vi "fail display.vi"(1 "P/F":bool[](array[boolean]), 2 "yellow":bool[](array[boolean]), 3 "Multipart board":cluster{"Row":i32, "Colum":i32}={"Row"=8, "Colum"=4}, 4 "colse":refnum<vi>) -> (0 "exit":bool=TRUE)   [LabVIEW 2018]
uses:
  <vilib>/Utility/miscctls.llb/LVBoundsTypeDef.ctl
  <vilib>/Utility/miscctls.llb/LVRowAndColumnTypeDef.ctl
panel:
  out "添加的数组":bool[][](array[boolean])
  out "数组 3":cluster{"Row":i32, "列":i32}[][](array[cluster])
  out "数组 2":cluster{"Row":i32, "列":i32}[](array[cluster])
  in  "F5":bool
  out "显示良品":u32(colorbox)=6618880
  out "显示不良品":u32(colorbox)=16711680
  out "数组":i32[][](array[numeric])
  out "输出簇 2":T1 caption="输出簇"
  out "输出簇":T1
  in  "表格控件":string[][](table)
  # "不良位置显示"
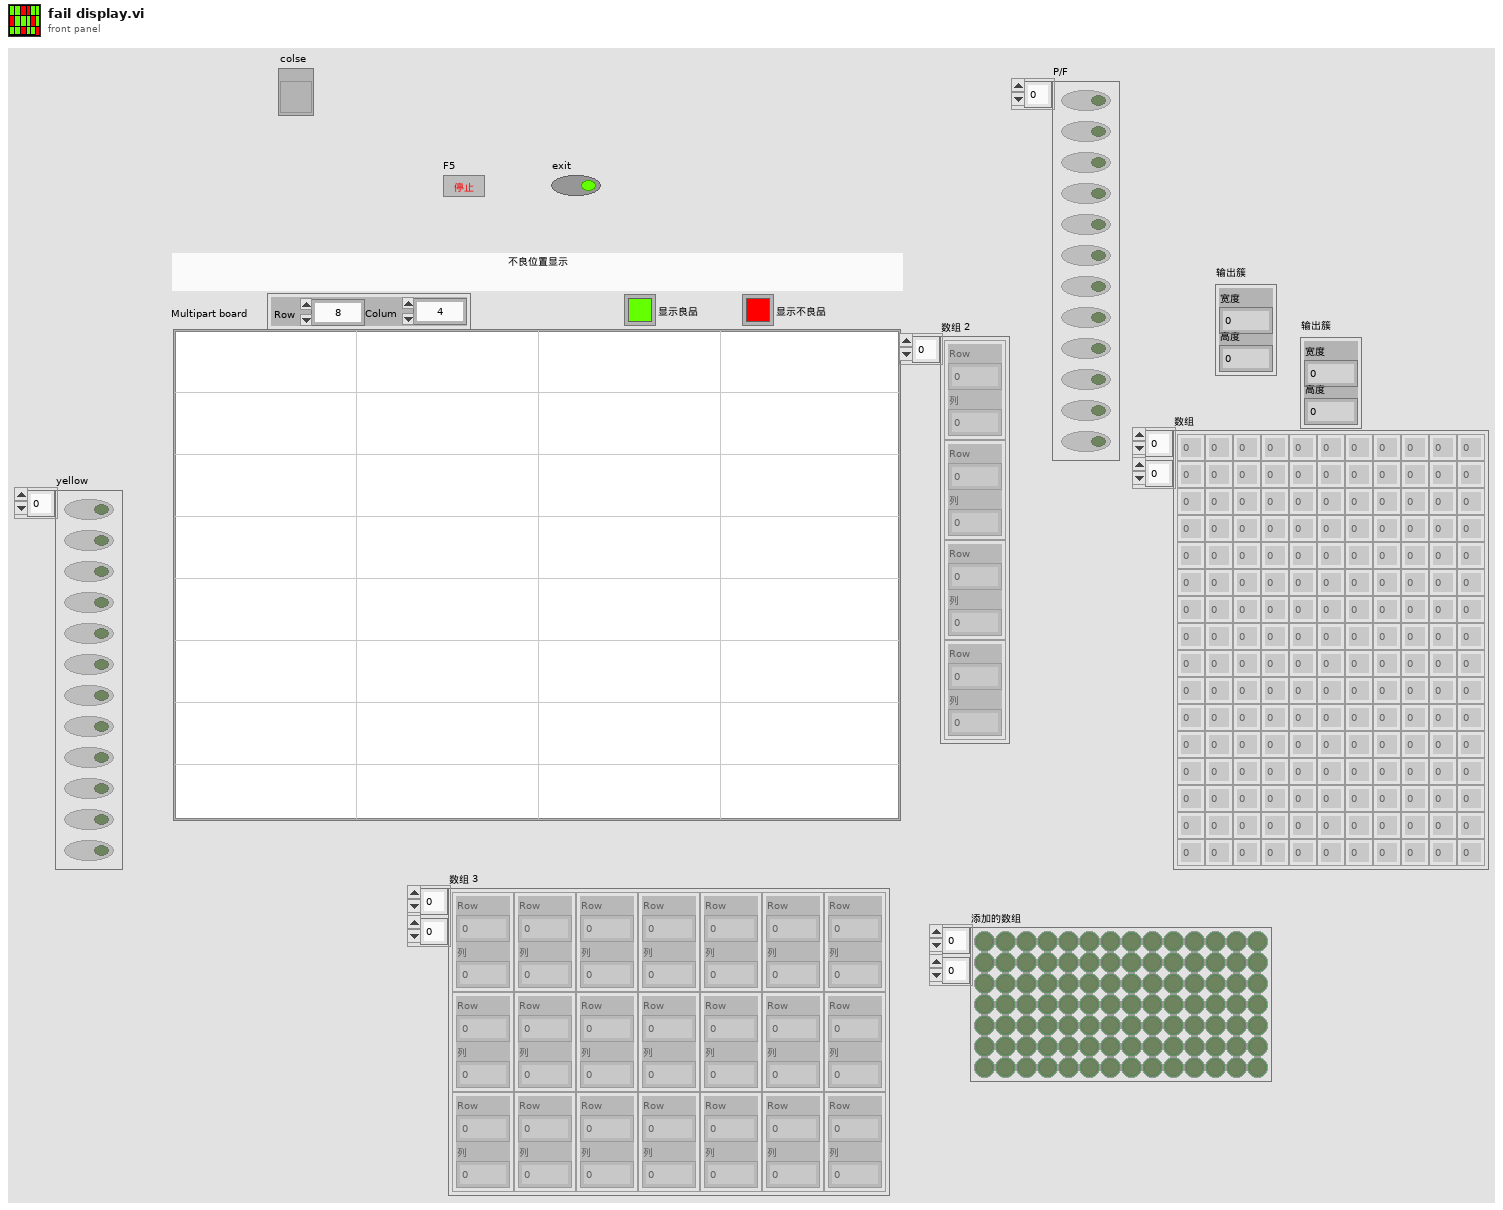
[diagram p1: front panel]
types:
  T1 = typedef "LVBoundsTypeDef.ctl" = cluster{"Width":u32, "Height":u32}
  T2 = typedef "LVRowAndColumnTypeDef.ctl" = cluster{"Row":i32, "Column":i32}
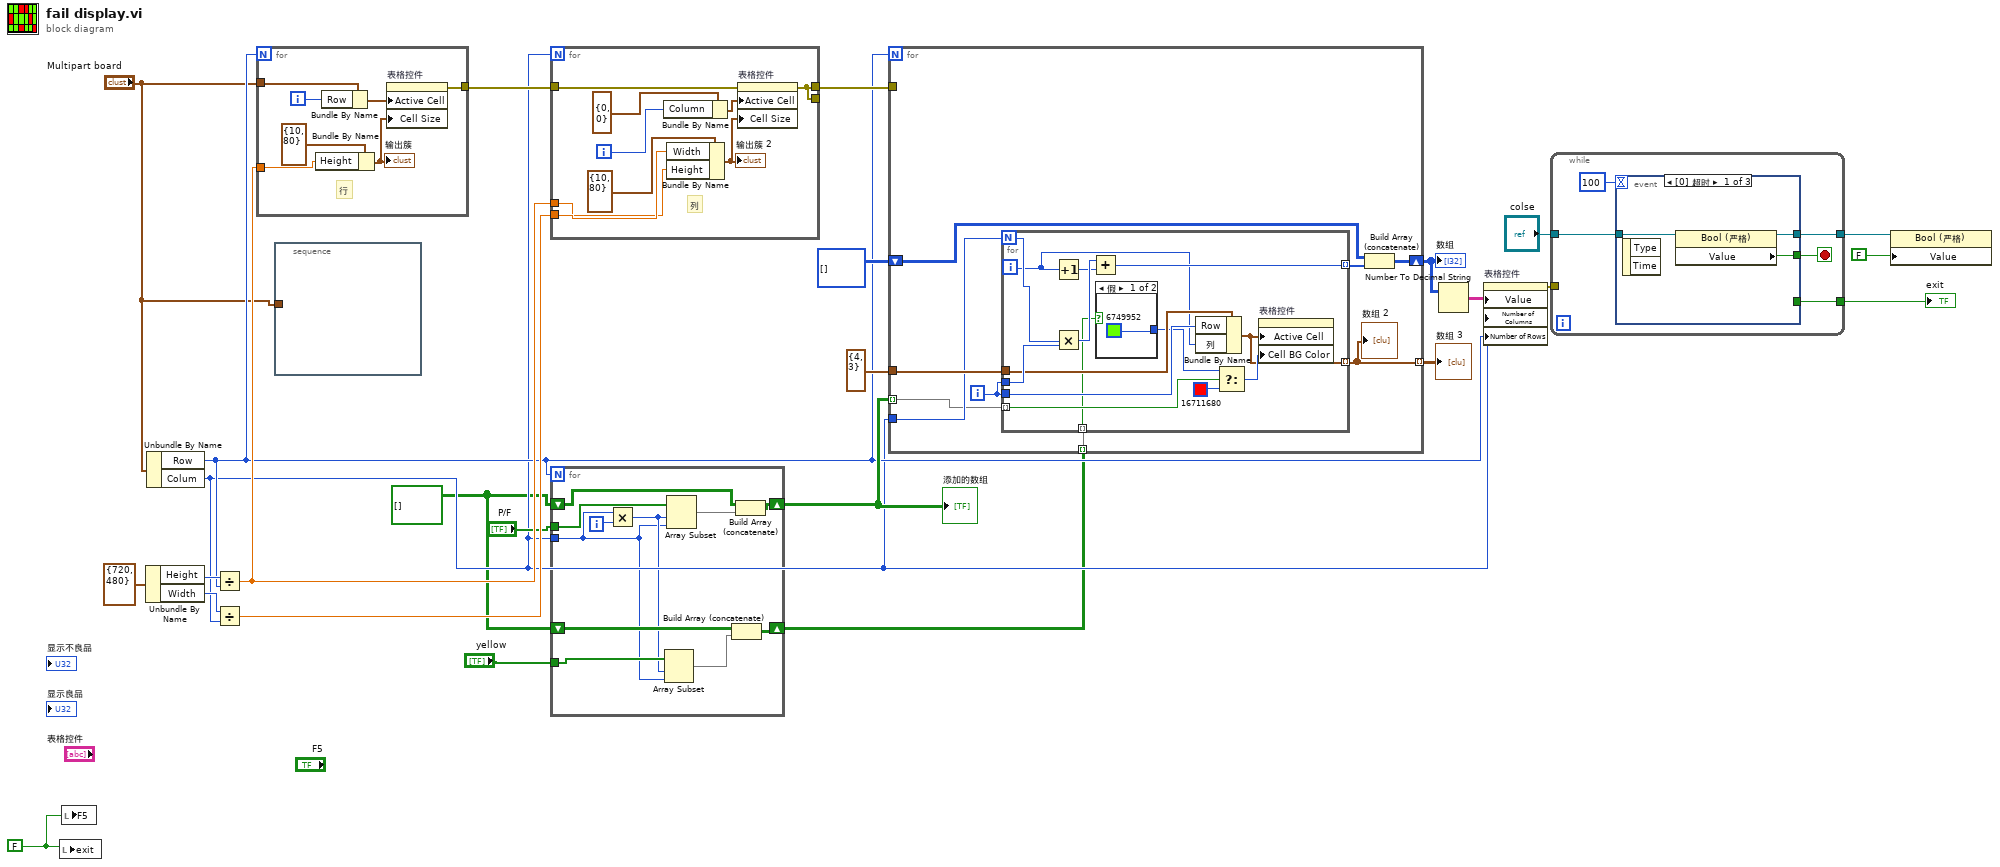
[diagram p0: block diagram]
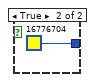
[diagram p2: hidden frame]
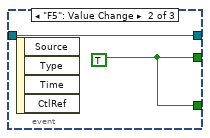
[diagram p3: hidden frame]
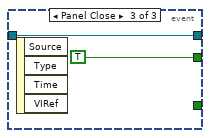
[diagram p4: hidden frame]
diagram:
  w1 = FALSE
  w6 = bool[][] [] ("添加的数组 2")
  n1 = local write "exit"(w1) -> ()
  n2 = local write "F5"(w1) -> ()
  n3 = Unbundle By Name(T1 {"Width"=720, "Height"=480} ("大小")) -> ("Height"=w18:u32, "Width"=w19:u32)
  n4 = Unbundle By Name("Multipart board") -> ("Row"=w9:i32, "Colum"=w8:i32)
  n5 = Divide(x=w18, y=w9) -> (x/y=w21:dbl)
  n6 = Divide(x=w19, y=w8) -> (x/y=w20:dbl)
  n7 = for {
    N: w9 -> [_]
    tunnel: w21 -> [w31]
    tunnel: [w29] -> w22
    tunnel: "Multipart board" -> [w27]
    i -> [w28]
    # "行"
    n8 = Bundle By Name(cluster=T1 {"Width"=10, "Height"=80} ("活动单元格:单元格大小"), "Height"=w31) -> (w30:T1)
    "输出簇" <- w30
    n9 = Bundle By Name(cluster=w27, "Row"=w28) -> (w33:cluster{"Row":i32, "Colum":i32})
    n10 = property on="表格控件" class="Tbl (严格)"("Active Cell"=w33, "Cell Size"=w30) -> (error out=w29:errorcluster)  [unwired: 2 in, 1 out]
  }
  n11 = stacked-sequence {
    tunnel: "Multipart board" -> [_]
    frame #0 {
    }
  }
  n12 = for {
    N: w8 -> [_]
    tunnel: w20 -> [w38]
    tunnel: w21 -> [w36]
    tunnel: w22 -> [w35]
    tunnel: [w34] -> _
    tunnel: [w34] -> w12
    i -> [w41]
    # "列"
    n13 = Bundle By Name(cluster=T2 {"Row"=0, "Column"=0} ("活动单元格:活动单元格"), "Column"=w41) -> (w42:T2)
    n14 = Bundle By Name(cluster=T1 {"Width"=10, "Height"=80} ("活动单元格:单元格大小"), "Width"=w38, "Height"=w36) -> (w37:T1)
    "输出簇 2" <- w37
    n15 = property on="表格控件" class="Tbl (严格)"(error in=w35, "Active Cell"=w42, "Cell Size"=w37) -> (error out=w34:errorcluster)  [unwired: 1 in, 1 out]
  }
  n16 = for {
    N: w9 -> [_]
    shift-right: [w51] -> w10
    shift-left: w6 -> [w52]
    tunnel: "P/F" -> [w53]
    tunnel: w8 -> [w43]
    tunnel: "yellow" -> [w46]
    shift-right: [w47] -> w4
    shift-left: w6 -> [w48]
    i -> [w49]
    n17 = Multiply(x=w43, y=w49) -> (x*y=w44:i32)
    n18 = Array Subset(array=w46, index=w44, length=w43) -> (w45:bool[])
    n19 = Array Subset(array=w53, index=w44, length=w43) -> (w50:bool[])
    n20 = Build Array (concatenate)(w48, w45) -> (w47:bool[][])
    n21 = Build Array (concatenate)(w52, w50) -> (w51:bool[][])
  }
  "添加的数组" <- w10
  n22 = for {
    N: w9 -> [_]
    shift-right: [w61] -> w24
    shift-left: i32[][] [] -> [w62]
    tunnel: w8 -> [w58]
    tunnel: cluster{"Row":i32, "列":i32} {"Row"=4, "列"=3} ("多联板 2") -> [w59]
    tunnel: w10 -> [w56] mode=indexing
    tunnel: [w55] -> w13 mode=indexing
    tunnel: w12 -> [_]
    tunnel: w4 -> [w54] mode=indexing
    i -> [w57]
    n23 = for {
      N: w58 -> [w75]
      tunnel: [w76] -> w60 mode=indexing
      tunnel: w57 -> [w74]
      tunnel: w59 -> [w71]
      tunnel: w57 -> [w69]
      tunnel: w56 -> [w68] mode=indexing
      tunnel: [w67] -> w55 mode=indexing
      tunnel: w54 -> [w63] mode=indexing
      i -> [w65]
      n24 = Increment(x=w65) -> (x+1=w72:i32)
      n25 = Multiply(x=w75, y=w74) -> (x*y=w73:i32)
      n26 = Add(x=w73, y=w72) -> (x+y=w76:i32)
      n27 = case shown="假" w63 {
        tunnel: [u32 6749952 u32 16776704] -> w64
        frame False {
        }
        frame True {
        }
      }
      n28 = Bundle By Name(cluster=w71, "Row"=w69, "列"=w65) -> (w67:cluster{"Row":i32, "列":i32})
      n29 = Select(t=w64, s=w68, f=u32 16711680) -> (s? t:f=w70:u32)
      n30 = property on="表格控件" class="Tbl (严格)"("Active Cell"=w67, "Cell BG Color"=w70) -> ()  [unwired: 2 in, 2 out]
    }
    "数组 2" <- w55
    n31 = Build Array (concatenate)(w62, w60) -> (w61:i32[][])
  }
  "数组" <- w24
  "数组 3" <- w13
  n32 = Number To Decimal String(number=w24) -> (decimal integer string=w25:string[][])  [unwired: 1 out]
  n33 = property on="表格控件" class="Tbl (严格)"("Value"=w25, "Number of Columns"=w8, "Number of Rows"=w9) -> (error out=w16:errorcluster)  [unwired: 2 in, 1 out]
  n34 = while {
    tunnel: "colse" -> [w83]
    tunnel: [w80] -> w14
    tunnel: w16 -> [_]
    tunnel: [w79] -> w3
    stop <- w82 stop-if-true
    n35 = event shown="[0] 超时" {
      selector: _ -> [_ _ _]
      dyn-events: _ -> [_ _ _]
      timeout: 100 -> [_ _ _]
      tunnel: w83 -> [w86 w87 w90]
      tunnel: [w84 w88 TRUE ("Value")] -> w82
      tunnel: [w85 w87 w90] -> w80
      tunnel: [_ w88 _] -> w79
      event Timeout {
        n36 = event-data() -> ()  [unwired: 3 out]
        n37 = property class="Bool (严格)"(reference=w86) -> (reference out=w85:refnum<vi>, "Value"=w84:bool)  [unwired: 1 in, 1 out]
      }
      event "F5": Value Change {
        w88 = TRUE
        n38 = event-data() -> ()  [unwired: 5 out]
      }
      event Panel Close {
        n39 = event-data() -> ()  [unwired: 5 out]
      }
    }
  }
  "exit" <- w3
  n40 = property class="Bool (严格)"(reference=w14, "Value"=FALSE) -> ()  [unwired: 1 in, 2 out]
